vi "read_ini.vi"(8 "error in (no error)":errorcluster caption="错误输入（无错误）", 9 "section name":string, 10 "file ref in":T1, 11 "StepMotor 输入":refnum<class "StepMotor.lvclass">) -> (0 "error out":errorcluster caption="错误输出", 2 "file ref out":T1, 3 "StepMotor 输出":refnum<class "StepMotor.lvclass">)   [LabVIEW 2016, in "MotionControl.lvlib" / "StepMotor.lvclass"]
uses:
  <userlib>/MotionControl/StepMotor/StepMotor.lvclass
  <vilib>/Utility/config.llb/Config Data RefNum.ctl
  <userlib>/MotionControl/StepMotor/StepMotor.lvclass/StepMotor.ctl
  <vilib>/Utility/config.llb/Read Key (I32).vi
  <vilib>/Utility/config.llb/Read Key (Double).vi
  <vilib>/Utility/config.llb/Read Key (U32).vi
  <vilib>/Utility/config.llb/Read Key (Boolean).vi
  <vilib>/ErrorRing/Error Ring.xnode
  <vilib>/Utility/config.llb/NI_LVConfig.lvlib
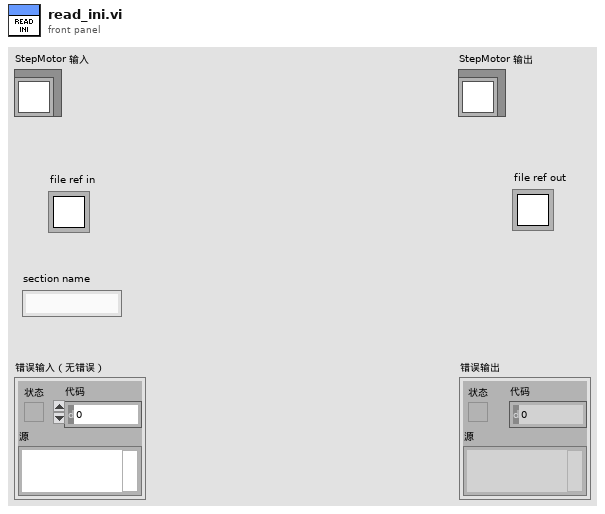
[diagram p1: front panel]
types:
  T1 = typedef "NI_LVConfig.lvlib/Config Data RefNum.ctl" = refnum<k1>
  T2 = typedef "MotionControl.lvlib/StepMotor.lvclass/AdvMovePara.ctl" = cluster{"acceleration":i32, "deceleration":i32, "max startup speed":i32, "max stop speed":i32}
  T3 = typedef "MotionControl.lvlib/StepMotor.lvclass/UIM_ICFG.ctl" = cluster{"ENA-开机自动使能":bool, "CCW-设置电机正转向":bool, "UPG-上电自动执行用户程序":bool, "ELOCK-紧急上锁功能":bool, "S1C-开机使能S1":bool, "S2C-开机使能S2":bool, "S3C-开机使能S3":bool, "S4C-开机使能S4":bool}
  T4 = typedef "MotionControl.lvlib/StepMotor.lvclass/UIM_MCFG.ctl" = cluster{"bS1IE":bool, "bS2IE":bool, "bS3IE":bool, "bP4IE":bool, "bSTPIE":bool, "bORGIE":bool, "bSTLIE":bool, "bDM":bool, "bAM":bool, "bCM":bool, "bQEM":bool, "bQEI":bool, "bCHS":bool, "bANE":bool}
  T5 = typedef "MotionControl.lvlib/StepMotor.lvclass/S12CON.ctl" = cluster{"S2传感器上升沿绑定动作":u32, "S2传感器下降沿绑定动作":u32, "S1传感器上升沿绑定动作":u32, "S1传感器下降沿绑定动作":u32}
  T6 = typedef "MotionControl.lvlib/StepMotor.lvclass/S34CON.ctl" = cluster{"TRUE: P4 出低电平; FALSE: P4 出高电平。":bool, "P4输出关联的事件代码":u32, "S3传感器上升沿绑定动作":u32, "S3传感器下降沿绑定动作":u32, "当发生堵转时动作":u32}
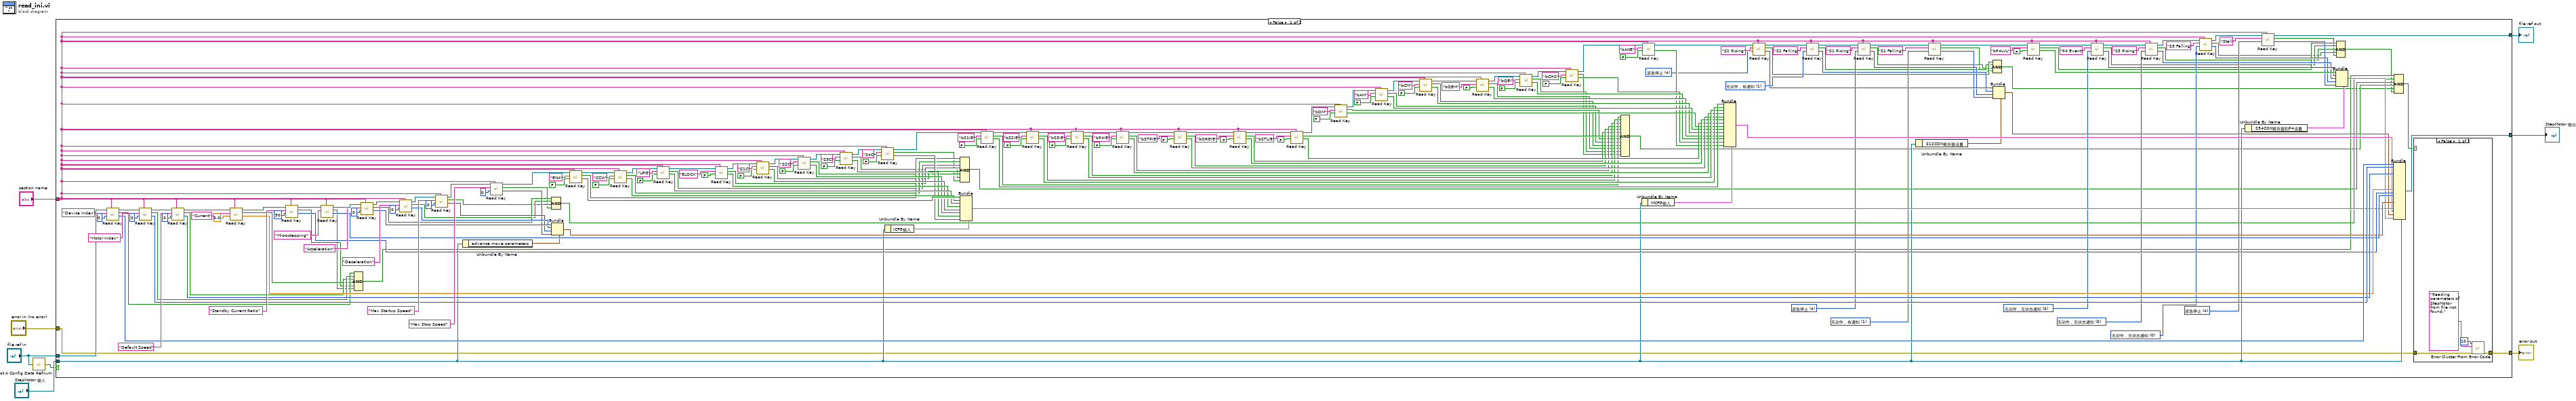
[diagram p0: block diagram]
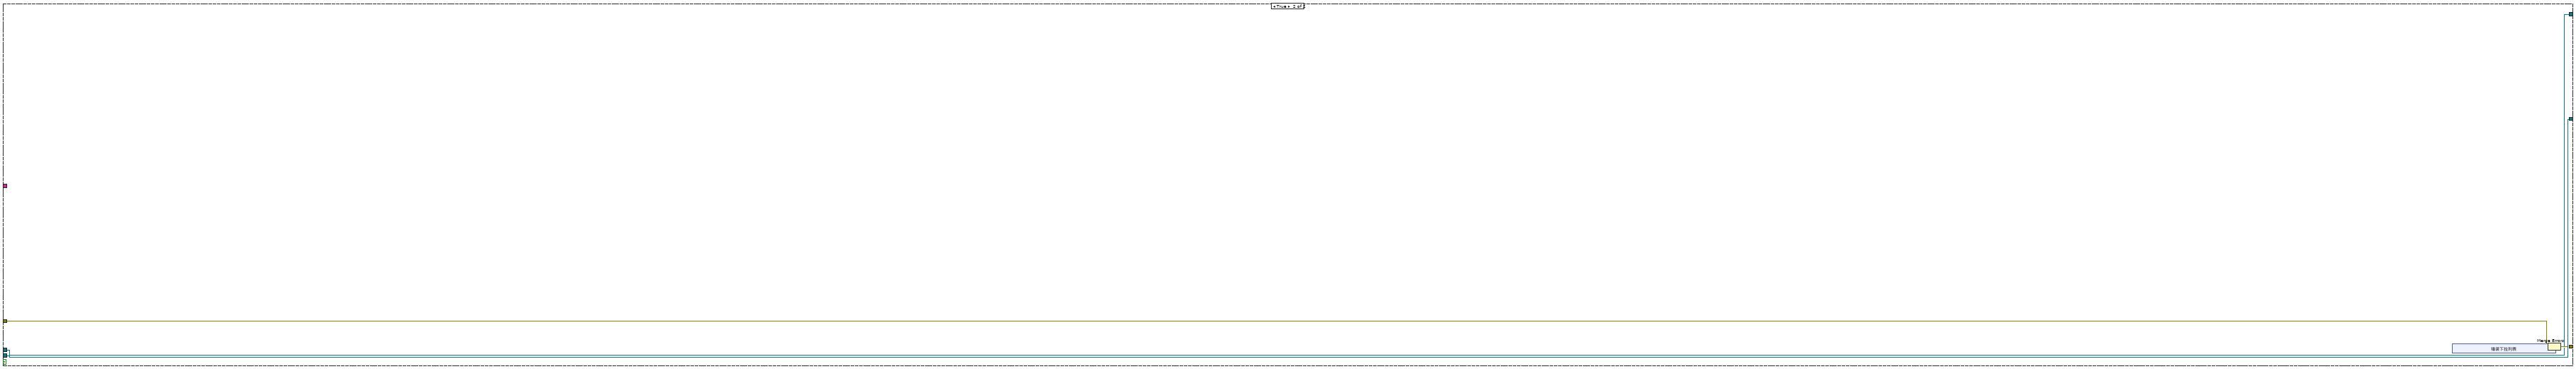
[diagram p3: hidden frame]
diagram:
  n1 = call <vilib>:"Not A Config Data Refnum.vi"("refnum"="file ref in") -> ("not a config data refnum"=w5:bool)
  n2 = case shown="False" w5 {
    tunnel: [w9 w241] -> w8
    tunnel: [w58 w244] -> w6
    tunnel: "StepMotor 输入" -> [w59 w244]
    tunnel: "error in (no error)" -> [w10 w242]
    tunnel: "section name" -> [w234 _]
    tunnel: "file ref in" -> [w233 w240]
    tunnel: [w232 w240] -> w1
    frame False {
      w64 = u32 4 items=["无动作，无状态通知", "无动作，有通知", "负向连续运行", "减速直到停止", "紧急停止", "负向相对位移控制", "绝对位置清零", "绝对位置清零+相对位移控制", "", "换向相对位移控制", "正向连续运行", "绝对位置清零+减速直到停止", "绝对位置清零+紧急停止", "正向相对位移控制", "换向连续运行", "脱机"] ("当发生堵转时动作")
      w65 = u32 0 items=["无动作，无状态通知"=0, "无动作，有通知"=1, "负向连续运行"=2, "减速直到停止"=3, "紧急停止"=4, "负向相对位移控制"=5, "绝对位置清零"=6, "绝对位置清零+相对位移控制"=7, "换向相对位移控制"=9, "正向连续运行"=10, "绝对位置清零+减速直到停止"=11, "绝对位置清零+紧急停止"=12, "正向相对位移控制"=13, "换向连续运行"=14, "脱机"=15] ("S3传感器下降沿绑定动作")
      w66 = u32 0 items=["无动作，无状态通知"=0, "无动作，有通知"=1, "负向连续运行"=2, "减速直到停止"=3, "紧急停止"=4, "负向相对位移控制"=5, "绝对位置清零"=6, "绝对位置清零+相对位移控制"=7, "换向相对位移控制"=9, "正向连续运行"=10, "绝对位置清零+减速直到停止"=11, "绝对位置清零+紧急停止"=12, "正向相对位移控制"=13, "换向连续运行"=14, "脱机"=15] ("S3传感器上升沿绑定动作")
      w67 = u32 0 items=["无动作，无状态通知", "电机转动，P4=指定电平；反之，P4相反", "电机正转，P4=指定电平；反之，P4相反", "位移大于等于0，P4=指定电平；反之，P4相反"] ("P4输出关联的事件代码")
      w77 = u32 1 items=["无动作，无状态通知"=0, "无动作，有通知"=1, "负向连续运行"=2, "减速直到停止"=3, "紧急停止"=4, "负向相对位移控制"=5, "绝对位置清零"=6, "绝对位置清零+相对位移控制"=7, "换向相对位移控制"=9, "正向连续运行"=10, "绝对位置清零+减速直到停止"=11, "绝对位置清零+紧急停止"=12, "正向相对位移控制"=13, "换向连续运行"=14, "脱机"=15] ("S1传感器下降沿绑定动作")
      w78 = u32 4 items=["无动作，无状态通知"=0, "无动作，有通知"=1, "负向连续运行"=2, "减速直到停止"=3, "紧急停止"=4, "负向相对位移控制"=5, "绝对位置清零"=6, "绝对位置清零+相对位移控制"=7, "换向相对位移控制"=9, "正向连续运行"=10, "绝对位置清零+减速直到停止"=11, "绝对位置清零+紧急停止"=12, "正向相对位移控制"=13, "换向连续运行"=14, "脱机"=15] ("S1传感器上升沿绑定动作")
      w79 = u32 1 items=["无动作，无状态通知"=0, "无动作，有通知"=1, "负向连续运行"=2, "减速直到停止"=3, "紧急停止"=4, "负向相对位移控制"=5, "绝对位置清零"=6, "绝对位置清零+相对位移控制"=7, "换向相对位移控制"=9, "正向连续运行"=10, "绝对位置清零+减速直到停止"=11, "绝对位置清零+紧急停止"=12, "正向相对位移控制"=13, "换向连续运行"=14, "脱机"=15] ("S2传感器下降沿绑定动作")
      w80 = u32 4 items=["无动作，无状态通知"=0, "无动作，有通知"=1, "负向连续运行"=2, "减速直到停止"=3, "紧急停止"=4, "负向相对位移控制"=5, "绝对位置清零"=6, "绝对位置清零+相对位移控制"=7, "换向相对位移控制"=9, "正向连续运行"=10, "绝对位置清零+减速直到停止"=11, "绝对位置清零+紧急停止"=12, "正向相对位移控制"=13, "换向连续运行"=14, "脱机"=15] ("S2传感器上升沿绑定动作")
      n3 = call-poly <vilib>:"Read Key.vi"("section"=w234, "default value"=0, "key"="Device Index", "refnum"=w233) -> ("value"=w150:i32, "found?"=w57:bool, "refnum out"=w216:T1)  [unwired: 4 in, 1 out]
      n4 = call-poly <vilib>:"Read Key.vi"("section"=w234, "default value"=0, "key"="Motor Index", "refnum"=w216) -> ("value"=w147:i32, "found?"=w56:bool, "refnum out"=w215:T1)  [unwired: 4 in, 1 out]
      n5 = call-poly <vilib>:"Read Key.vi"("section"=w234, "default value"=0, "key"="Default Speed", "refnum"=w215) -> ("value"=w145:i32, "found?"=w55:bool, "refnum out"=w230:T1)  [unwired: 4 in, 1 out]
      n6 = call-poly <vilib>:"Read Key.vi"("section"=w234, "default value"=0.0, "key"="Current", "refnum"=w230) -> ("value"=w143:dbl, "found?"=w54:bool, "refnum out"=w227:T1)  [unwired: 4 in, 1 out]
      n7 = call-poly <vilib>:"Read Key.vi"("section"=w234, "default value"=50, "key"="Standby Current Ratio", "refnum"=w227) -> ("value"=w141:i32, "found?"=w53:bool, "refnum out"=w225:T1)  [unwired: 4 in, 1 out]
      n8 = call-poly <vilib>:"Read Key.vi"("section"=w234, "key"="Microstepping", "refnum"=w225) -> ("value"=w140:u32, "found?"=w52:bool, "refnum out"=w224:T1)  [unwired: 5 in, 1 out]
      n9 = Compound Arithmetic op=AND(w57, w56, w55, w54, w53, w52) -> (w17:bool)
      n10 = call-poly <vilib>:"Read Key.vi"("section"=w234, "default value"=0, "key"="Acceleration", "refnum"=w224) -> ("value"=w138:i32, "found?"=w51:bool, "refnum out"=w222:T1)  [unwired: 4 in, 1 out]
      n11 = call-poly <vilib>:"Read Key.vi"("section"=w234, "default value"=0, "key"="Deceleration", "refnum"=w222) -> ("value"=w135:i32, "found?"=w50:bool, "refnum out"=w221:T1)  [unwired: 4 in, 1 out]
      n12 = call-poly <vilib>:"Read Key.vi"("section"=w234, "default value"=0, "key"="Max Startup Speed", "refnum"=w221) -> ("value"=w133:i32, "found?"=w49:bool, "refnum out"=w220:T1)  [unwired: 4 in, 1 out]
      n13 = Unbundle By Name(w59) -> ("advance move parameters"=w139:T2)
      n14 = call-poly <vilib>:"Read Key.vi"("section"=w234, "default value"=0, "key"="Max Stop Speed", "refnum"=w220) -> ("value"=w131:i32, "found?"=w48:bool, "refnum out"=w197:T1)  [unwired: 4 in, 1 out]
      n15 = Compound Arithmetic op=AND(w51, w50, w49, w48) -> (w16:bool)
      n16 = Bundle(cluster=w139, "acceleration"=w138, "deceleration"=w135, "max startup speed"=w133, "max stop speed"=w131) -> (w130:T2)
      n17 = call-poly <vilib>:"Read Key.vi"("section"=w234, "default value"=FALSE, "key"="ENA", "refnum"=w197) -> ("value"=w127:bool, "found?"=w47:bool, "refnum out"=w208:T1)  [unwired: 4 in, 1 out]
      n18 = call-poly <vilib>:"Read Key.vi"("section"=w234, "default value"=FALSE, "key"="CCW", "refnum"=w208) -> ("value"=w125:bool, "found?"=w46:bool, "refnum out"=w207:T1)  [unwired: 4 in, 1 out]
      n19 = call-poly <vilib>:"Read Key.vi"("section"=w234, "default value"=FALSE, "key"="UPG", "refnum"=w207) -> ("value"=w123:bool, "found?"=w45:bool, "refnum out"=w206:T1)  [unwired: 4 in, 1 out]
      n20 = call-poly <vilib>:"Read Key.vi"("section"=w234, "default value"=FALSE, "key"="ELOCK", "refnum"=w206) -> ("value"=w121:bool, "found?"=w44:bool, "refnum out"=w198:T1)  [unwired: 4 in, 1 out]
      n21 = call-poly <vilib>:"Read Key.vi"("section"=w234, "default value"=FALSE, "key"="S1C", "refnum"=w198) -> ("value"=w119:bool, "found?"=w43:bool, "refnum out"=w201:T1)  [unwired: 4 in, 1 out]
      n22 = call-poly <vilib>:"Read Key.vi"("section"=w234, "default value"=FALSE, "key"="S2C", "refnum"=w201) -> ("value"=w117:bool, "found?"=w42:bool, "refnum out"=w200:T1)  [unwired: 4 in, 1 out]
      n23 = call-poly <vilib>:"Read Key.vi"("section"=w234, "default value"=FALSE, "key"="S3C", "refnum"=w200) -> ("value"=w115:bool, "found?"=w41:bool, "refnum out"=w199:T1)  [unwired: 4 in, 1 out]
      n24 = call-poly <vilib>:"Read Key.vi"("section"=w234, "default value"=FALSE, "key"="S4C", "refnum"=w199) -> ("value"=w113:bool, "found?"=w40:bool, "refnum out"=w169:T1)  [unwired: 4 in, 1 out]
      n25 = Unbundle By Name(w59) -> ("ICFG输入"=w129:T3)
      n26 = Compound Arithmetic op=AND(w47, w46, w45, w44, w43, w42, w41, w40) -> (w15:bool)
      n27 = Bundle(cluster=w129, "ENA-开机自动使能"=w127, "CCW-设置电机正转向"=w125, "UPG-上电自动执行用户程序"=w123, "ELOCK-紧急上锁功能"=w121, "S1C-开机使能S1"=w119, "S2C-开机使能S2"=w117, "S3C-开机使能S3"=w115, "S4C-开机使能S4"=w113) -> (w112:T3)
      n28 = call-poly <vilib>:"Read Key.vi"("section"=w234, "default value"=FALSE, "key"="bS1IE", "refnum"=w169) -> ("value"=w96:bool, "found?"=w39:bool, "refnum out"=w192:T1)  [unwired: 4 in, 1 out]
      n29 = call-poly <vilib>:"Read Key.vi"("section"=w234, "default value"=FALSE, "key"="bS2IE", "refnum"=w192) -> ("value"=w95:bool, "found?"=w38:bool, "refnum out"=w191:T1)  [unwired: 4 in, 1 out]
      n30 = call-poly <vilib>:"Read Key.vi"("section"=w234, "default value"=FALSE, "key"="bS3IE", "refnum"=w191) -> ("value"=w94:bool, "found?"=w37:bool, "refnum out"=w190:T1)  [unwired: 4 in, 1 out]
      n31 = call-poly <vilib>:"Read Key.vi"("section"=w234, "default value"=FALSE, "key"="bP4IE", "refnum"=w190) -> ("value"=w93:bool, "found?"=w36:bool, "refnum out"=w172:T1)  [unwired: 4 in, 1 out]
      n32 = call-poly <vilib>:"Read Key.vi"("section"=w234, "default value"=FALSE, "key"="bSTPIE", "refnum"=w172) -> ("value"=w92:bool, "found?"=w35:bool, "refnum out"=w185:T1)  [unwired: 4 in, 1 out]
      n33 = call-poly <vilib>:"Read Key.vi"("section"=w234, "default value"=FALSE, "key"="bORGIE", "refnum"=w185) -> ("value"=w91:bool, "found?"=w34:bool, "refnum out"=w184:T1)  [unwired: 4 in, 1 out]
      n34 = call-poly <vilib>:"Read Key.vi"("section"=w234, "default value"=FALSE, "key"="bSTLIE", "refnum"=w184) -> ("value"=w90:bool, "found?"=w33:bool, "refnum out"=w183:T1)  [unwired: 4 in, 1 out]
      n35 = call-poly <vilib>:"Read Key.vi"("section"=w234, "default value"=FALSE, "key"="bDM", "refnum"=w183) -> ("value"=w89:bool, "found?"=w32:bool, "refnum out"=w171:T1)  [unwired: 4 in, 1 out]
      n36 = call-poly <vilib>:"Read Key.vi"("section"=w234, "default value"=FALSE, "key"="bAM", "refnum"=w171) -> ("value"=w88:bool, "found?"=w31:bool, "refnum out"=w178:T1)  [unwired: 4 in, 1 out]
      n37 = call-poly <vilib>:"Read Key.vi"("section"=w234, "default value"=FALSE, "key"="bCM", "refnum"=w178) -> ("value"=w87:bool, "found?"=w30:bool, "refnum out"=w177:T1)  [unwired: 4 in, 1 out]
      n38 = call-poly <vilib>:"Read Key.vi"("section"=w234, "default value"=FALSE, "key"="bQEM", "refnum"=w177) -> ("value"=w86:bool, "found?"=w29:bool, "refnum out"=w176:T1)  [unwired: 4 in, 1 out]
      n39 = call-poly <vilib>:"Read Key.vi"("section"=w234, "default value"=FALSE, "key"="bQEI", "refnum"=w176) -> ("value"=w85:bool, "found?"=w28:bool, "refnum out"=w170:T1)  [unwired: 4 in, 1 out]
      n40 = call-poly <vilib>:"Read Key.vi"("section"=w234, "default value"=FALSE, "key"="bCHS", "refnum"=w170) -> ("value"=w84:bool, "found?"=w27:bool, "refnum out"=w173:T1)  [unwired: 4 in, 1 out]
      n41 = Compound Arithmetic op=AND(w39, w38, w37, w36, w35, w34, w33, w32, w31, w30, w29, w28, w27) -> (w14:bool)
      n42 = Unbundle By Name(w59) -> ("MCFG输入"=w111:T4)
      n43 = call-poly <vilib>:"Read Key.vi"("section"=w234, "default value"=FALSE, "key"="bANE", "refnum"=w173) -> ("value"=w83:bool, "refnum out"=w154:T1)  [unwired: 4 in, 2 out]
      n44 = Bundle(cluster=w111, "bS1IE"=w96, "bS2IE"=w95, "bS3IE"=w94, "bP4IE"=w93, "bSTPIE"=w92, "bORGIE"=w91, "bSTLIE"=w90, "bDM"=w89, "bAM"=w88, "bCM"=w87, "bQEM"=w86, "bQEI"=w85, "bCHS"=w84, "bANE"=w83) -> (w82:T4)
      n45 = call-poly <vilib>:"Read Key.vi"("section"=w234, "default value"=w80, "key"="S2 Rising", "refnum"=w154) -> ("value"=w76:u32, "found?"=w26:bool, "refnum out"=w164:T1)  [unwired: 4 in, 1 out]
      n46 = call-poly <vilib>:"Read Key.vi"("section"=w234, "default value"=w79, "key"="S2 Falling", "refnum"=w164) -> ("value"=w75:u32, "found?"=w25:bool, "refnum out"=w163:T1)  [unwired: 4 in, 1 out]
      n47 = call-poly <vilib>:"Read Key.vi"("section"=w234, "default value"=w78, "key"="S1 Rising", "refnum"=w163) -> ("value"=w74:u32, "found?"=w24:bool, "refnum out"=w162:T1)  [unwired: 4 in, 1 out]
      n48 = Unbundle By Name(w59) -> ("S12CON寄存器设置"=w81:T5)
      n49 = call-poly <vilib>:"Read Key.vi"("section"=w234, "default value"=w77, "key"="S1 Falling", "refnum"=w162) -> ("value"=w73:u32, "found?"=w23:bool, "refnum out"=w151:T1)  [unwired: 4 in, 1 out]
      n50 = Compound Arithmetic op=AND(w26, w25, w24, w23) -> (w13:bool)
      n51 = Bundle(cluster=w81, "S2传感器上升沿绑定动作"=w76, "S2传感器下降沿绑定动作"=w75, "S1传感器上升沿绑定动作"=w74, "S1传感器下降沿绑定动作"=w73) -> (w72:T5)
      n52 = call-poly <vilib>:"Read Key.vi"("section"=w234, "default value"=FALSE, "key"="bP4LVL", "refnum"=w151) -> ("value"=w68:bool, "found?"=w22:bool, "refnum out"=w157:T1)  [unwired: 4 in, 1 out]
      n53 = call-poly <vilib>:"Read Key.vi"("section"=w234, "default value"=w67, "key"="P4 Event", "refnum"=w157) -> ("value"=w63:u32, "found?"=w21:bool, "refnum out"=w156:T1)  [unwired: 4 in, 1 out]
      n54 = call-poly <vilib>:"Read Key.vi"("section"=w234, "default value"=w66, "key"="S3 Rising", "refnum"=w156) -> ("value"=w62:u32, "found?"=w20:bool, "refnum out"=w155:T1)  [unwired: 4 in, 1 out]
      n55 = call-poly <vilib>:"Read Key.vi"("section"=w234, "default value"=w65, "key"="S3 Falling", "refnum"=w155) -> ("value"=w61:u32, "found?"=w19:bool, "refnum out"=w152:T1)  [unwired: 4 in, 1 out]
      n56 = Unbundle By Name(w59) -> ("S34CON寄存器和P4设置"=w70:T6)
      n57 = call-poly <vilib>:"Read Key.vi"("section"=w234, "default value"=w64, "key"="Stall", "refnum"=w152) -> ("value"=w60:u32, "found?"=w18:bool, "refnum out"=w232:T1)  [unwired: 4 in, 1 out]
      n58 = Bundle(cluster=w70, "TRUE: P4 出低电平; FALSE: P4 出高电平。"=w68, "P4输出关联的事件代码"=w63, "S3传感器上升沿绑定动作"=w62, "S3传感器下降沿绑定动作"=w61, "当发生堵转时动作"=w60) -> (w69:T6)
      n59 = Compound Arithmetic op=AND(w22, w21, w20, w19, w18) -> (w12:bool)
      n60 = Bundle(cluster=w59, w150, w147, w145, w143, w141, w140, w130, w112, w82, w72, w69) -> (w58:refnum<class "StepMotor.lvclass">)  [unwired: 7 in]
      n61 = Compound Arithmetic op=AND(w17, w16, w15, w14, w13, w12) -> (w11:bool)
      n62 = case shown="False" w11 {
        tunnel: w10 -> [w236 w239]
        tunnel: [w235 w239] -> w9
        frame False {
          n63 = call <vilib>:"Error Cluster From Error Code.vi"("error in (no error)"=w236, "error message (\"\")"="Reading parameters of StepMotor from file not found." ("error message (\"\")"), "error code (0)"=10) -> ("error out"=w235:errorcluster)  [unwired: 6 in]
        }
        frame True {
        }
      }
    }
    frame True {
      n64 = xnode "错误下拉列表"() -> ("error out"=w243:errorcluster)
      n65 = Merge Errors(w242, w243) -> (w241:errorcluster)
    }
  }
  "error out" <- w8
  "StepMotor 输出" <- w6
  "file ref out" <- w1
